vi "LINC Scale Polynomial.vi"(1 "poly scale":cluster{"coefficients":dbl[]}[](array[cluster]), 2 "poly bounds":dbl[](array[numeric]), 3 "unscaled value":dbl) -> (0 "scaled value":dbl)   [LabVIEW 2018, in "STEPkgDriver_LINC.lvlib"]
uses:
  STEPkgDriver_LINC.lvlib
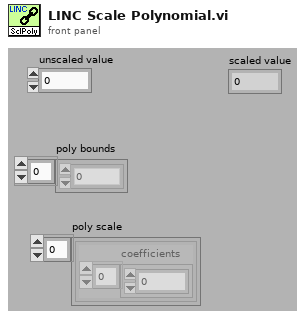
[diagram p1: front panel]
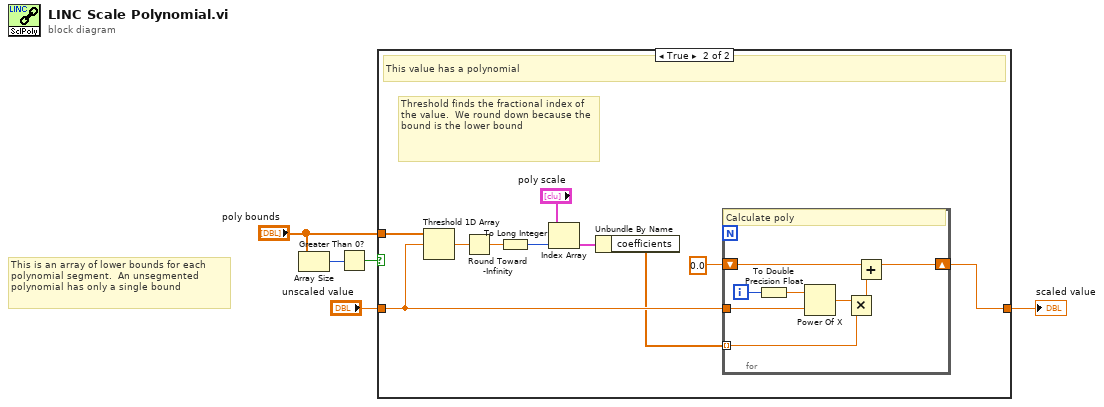
[diagram p0: block diagram]
diagram:
  # "This is an array of lower bounds for each polynomial segment.  An unsegmented polynomial has only a single bound"
  n1 = Array Size(array="poly bounds") -> (size(s)=w2:i32)
  n2 = Greater Than 0?(x=w2) -> (x > 0?=w1:bool)
  n3 = case shown="True" w1 {
    tunnel: "unscaled value" -> [w6 w11]
    tunnel: "poly bounds" -> [_ w12]
    tunnel: [w6 w15] -> w4
    frame False {
      # "No polynomial.  Do nothing"
    }
    frame True {
      # "Threshold finds the fractional index of the value.  We round down because the bound is the lower bound"
      # "This value has a polynomial"
      n4 = Threshold 1D Array(2:w11, 3:w12) -> (0:w14:dbl)  [unwired: 1 in]
      n5 = Round Toward -Infinity(1:w14) -> (0:w13:dbl)
      n6 = To Long Integer(number=w13) -> (32bit integer=w10:i32)
      n7 = Index Array(array="poly scale", index=w10) -> (element=w8:cluster{"coefficients":dbl[]})
      n8 = Unbundle By Name(w8) -> ("coefficients"=w7:dbl[])
      n9 = for {
        tunnel: w11 -> [w22]
        tunnel: w7 -> [w20] mode=indexing
        shift-right: [w17] -> w15
        shift-left: 0.0 -> [w19]
        i -> [w24]
        # "Calculate poly"
        n10 = To Double Precision Float(number=w24) -> (double precision float=w23:dbl)
        n11 = Power Of X(1:w22, 2:w23) -> (0:w21:dbl)
        n12 = Multiply(x=w21, y=w20) -> (x*y=w18:dbl)
        n13 = Add(x=w19, y=w18) -> (x+y=w17:dbl)
      }
    }
  }
  "scaled value" <- w4
